vi "FixNames.vi"(1 "name":string) -> (0 "python name":string)   [LabVIEW 2014, in "Python Functions.lvlib"]
uses:
  Python Functions.lvlib
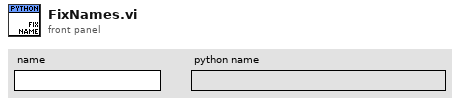
[diagram p1: front panel]
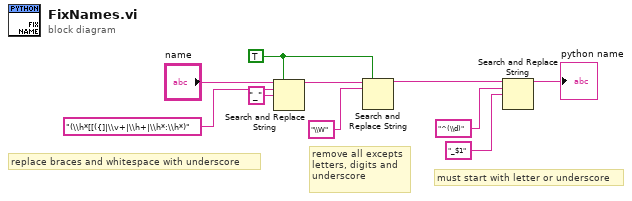
[diagram p0: block diagram]
diagram:
  w6 = TRUE ("replace all? (F)")
  # "must start with letter or underscore"
  # "remove all excepts\nletters, digits and \nunderscore"
  # "replace braces and whitespace with underscore"
  n1 = Search and Replace String(replace all?=w6, input string="name", search string="(\\h*[[({]|\\v+|\\h+|\\h*:\\h*)", replace string="_" ("replace string (\"\")")) -> (result string=w7:string)  [unwired: 4 in, 3 out]
  n2 = Search and Replace String(replace all?=w6, input string=w7, search string="\\W") -> (result string=w4:string)  [unwired: 5 in, 3 out]
  n3 = Search and Replace String(input string=w4, search string="^(\\d)", replace string="_$1" ("replace string (\"\")")) -> (result string=→"python name":string)  [unwired: 5 in, 3 out]
